vi "Check position limit.vi"(10 "Move By":dbl, 11 "Status in":T1) -> (2 "In range":bool)   [LabVIEW 2017]
uses:
  ctl/Servo state.ctl
  ctl/Servo variables.ctl
  ctl/Servo constants.ctl
  ctl/Axis names.ctl
  Servo drive module.lvlib
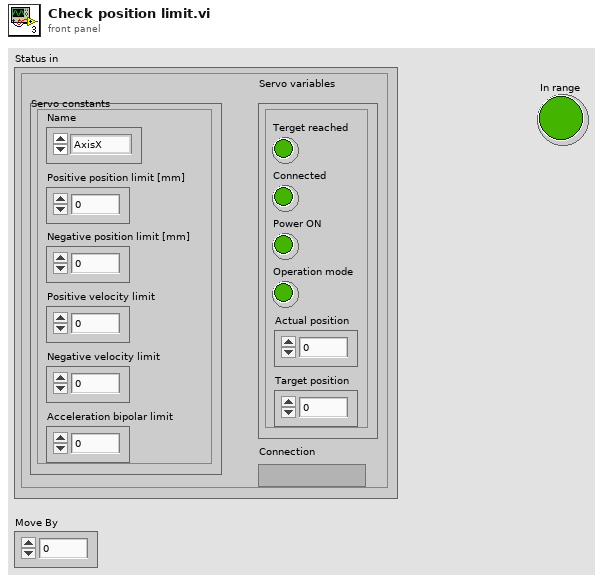
[diagram p1: front panel]
types:
  T1 = typedef "Servo drive module.lvlib/Servo state.ctl" = cluster{"Servo variables":T2, "Servo constants":T3, "Connection":variant}
  T2 = typedef "Servo drive module.lvlib/Servo variables.ctl" = cluster{"Terget reached":bool, "Connected":bool, "Power ON":bool, "Operation mode":bool, "Actual position":dbl, "Target position":dbl}
  T3 = typedef "Servo drive module.lvlib/Servo constants.ctl" = cluster{"Name":T4, "Positive position limit [mm]":dbl, "Negative position limit [mm]":dbl, "Positive velocity limit":dbl, "Negative velocity limit":dbl, "Acceleration bipolar limit":dbl}
  T4 = typedef "Servo drive module.lvlib/Axis names.ctl" = enum16{"AxisX", "AxisY", "AxisZ_left", "AxisZ_middle", "AxisZ_right"}
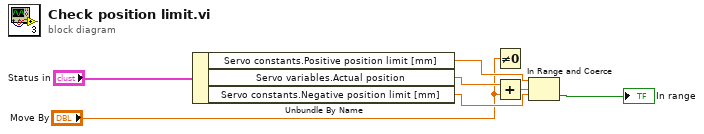
[diagram p0: block diagram]
diagram:
  n1 = Unbundle By Name("Status in") -> ("Servo constants.Positive position limit [mm]"=w3:dbl, "Servo variables.Actual position"=w4:dbl, "Servo constants.Negative position limit [mm]"=w5:dbl)
  n2 = Not Equal To 0?(x="Move By") -> ()  [unwired: 1 out]
  n3 = Add(x=w4, y="Move By") -> (x+y=w6:dbl)
  n4 = In Range and Coerce(upper limit=w3, x=w6, lower limit=w5) -> (In Range?=→"In range":bool)  [unwired: 1 out]
